vi "SendCmd.vi"(2 "索引 (行)":u8) -> (0 "字符串":string)   [LabVIEW 2011]
panel:
  # "发送命令函数子VI"
  # "进入DFTP模式"
  # "接收Sensor Data"
  # "接收Version Data"
  # "接收Sensor+Version Data"
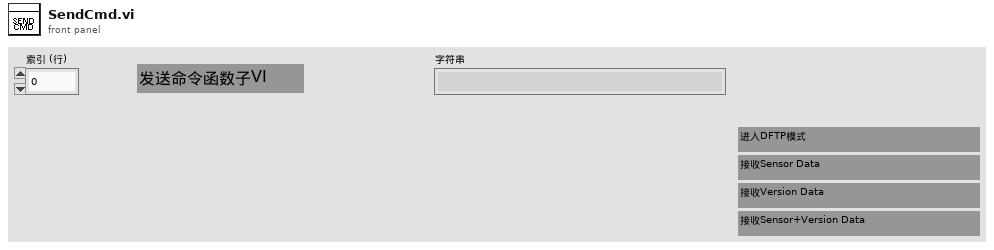
[diagram p1: front panel]
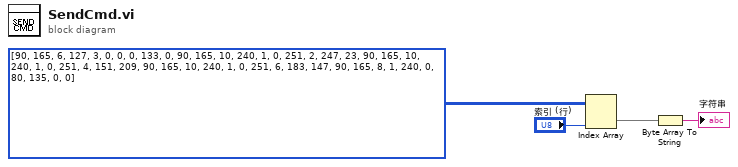
[diagram p0: block diagram]
diagram:
  n1 = Index Array(array=u8[][] [[90, 165, 6, 127, 3, 0, 0, 0, 133, 0], [90, 165, 10, 240, 1, 0, 251, 2, 247, 23], [90, 165, 10, 240, 1, 0, 251, 4, 151, 209], [90, 165, 10, 240, 1, 0, 251, 6, 183, 147], [90, 165, 8, 1, 240, 0, 80, 135, 0, 0]] ("mu08CmdArray"), index (row)="索引 (行)") -> (element=w3:u8[])  [unwired: 1 in]
  n2 = Byte Array To String(unsigned byte array=w3) -> (string=→"字符串":string)
